vi "as2_startLogFile.vi"(4 "error in (no error)":errorcluster, 6 "Path In":path) -> (0 "error out":errorcluster, 2 "Path":path)   [LabVIEW 2013]
uses:
  <vilib>/Utility/file.llb/Write To Spreadsheet File (string).vi
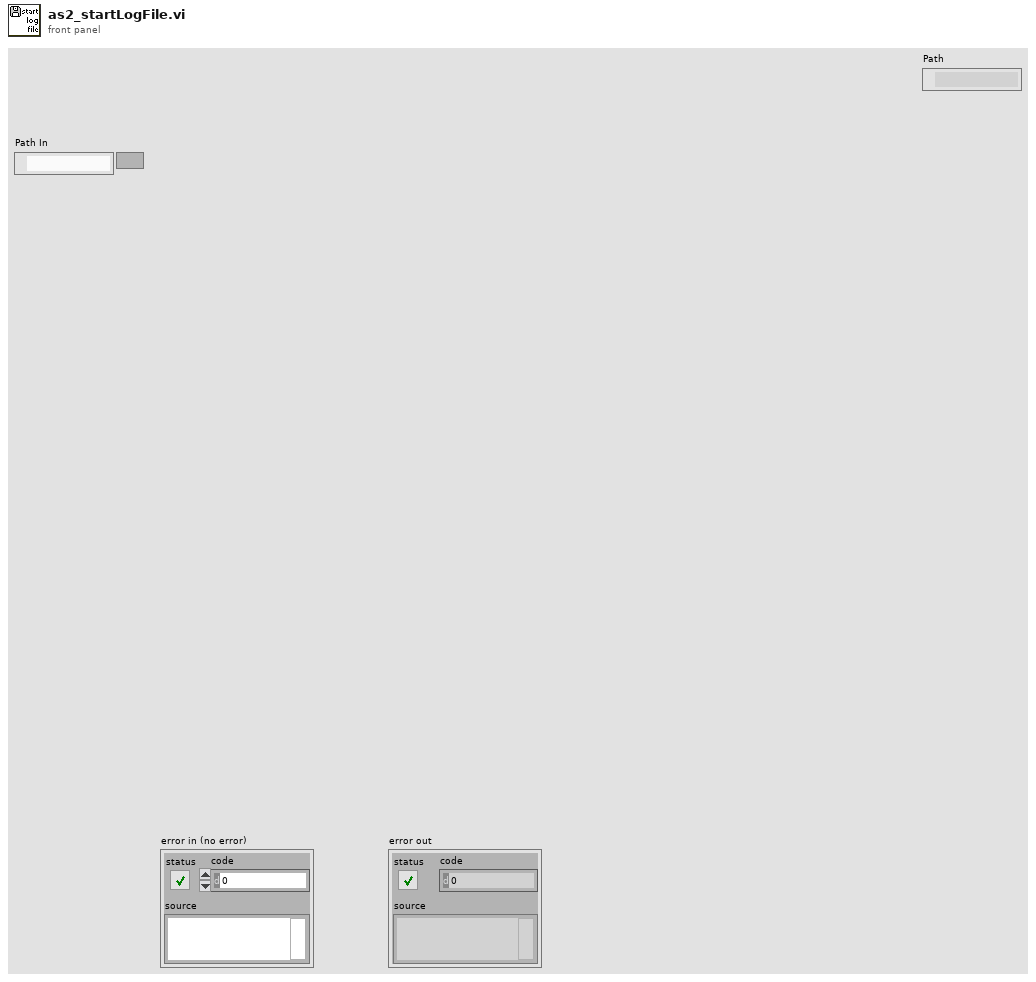
[diagram p1: front panel]
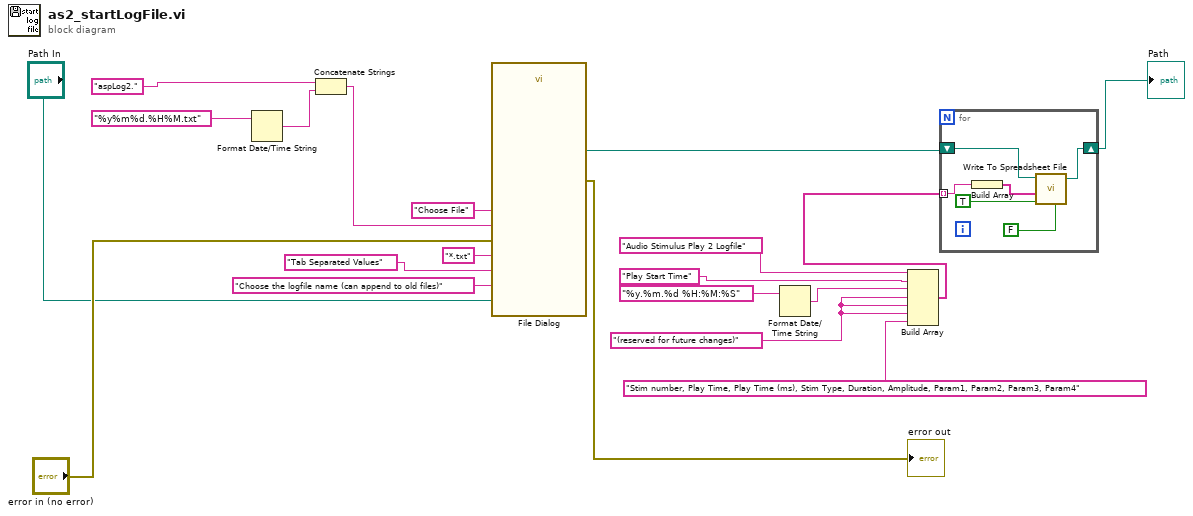
[diagram p0: block diagram]
diagram:
  w1 = "(reserved for future changes)" ("element")
  n1 = Format Date/Time String(time format string (%c)="%y%m%d.%H%M.txt") -> (date/time string=w15:string)  [unwired: 2 in]
  n2 = Concatenate Strings("aspLog2.", w15) -> (w14:string)
  n3 = call "File Dialog"("start path"="Path In", "prompt"="Choose the logfile name (can append to old files)", "button label"="Choose File", "default name"=w14, "error in"="error in (no error)", "pattern (all files)"="*.txt", "pattern label"="Tab Separated Values") -> ("selected path"=w4:path, "error out"=→"error out":errorcluster)  [unwired: 5 in, 2 out]
  n4 = Format Date/Time String(time format string (%c)="%y.%m.%d %H:%M:%S") -> (date/time string=w5:string)  [unwired: 2 in]
  n5 = Build Array("Audio Stimulus Play 2 Logfile", "Play Start Time", w5, w1, w1, w1, "Stim number, Play Time, Play Time (ms), Stim Type, Duration, Amplitude, Param1, Param2, Param3, Param4") -> (w6:string[])
  n6 = for {
    tunnel: w6 -> [w23] mode=indexing
    shift-right: [w25] -> w3
    shift-left: w4 -> [w24]
    n7 = Build Array(w23) -> (w22:string[])
    n8 = call-poly <vilib>:"Write To Spreadsheet File.vi"("transpose? (no:F)"=FALSE, "append to file? (new file:F)"=TRUE, "1D data"=w22, "file path (dialog if empty)"=w24) -> ("new file path (Not A Path if cancelled)"=w25:path)  [unwired: 4 in]
  }
  "Path" <- w3
